vi "WPI_SerialPortWrite.vi"(8 "error in (no error)":errorcluster, 10 "Buffer":string, 11 "SerialPortRef":T1) -> (0 "error out":errorcluster, 2 "Num Bytes Written":u32, 3 "SerialPortRef":T1)   [LabVIEW 2017]
doc: "Writes data to the serial device you specify.\n\nThis software is licensed. Open the labview\\readme\\WPI Robotics Library Open Source License.txt file for more information."
uses:
  <vilib>/Rock Robotics/WPI/SerialPort/WPI_SerialPortRef.ctl
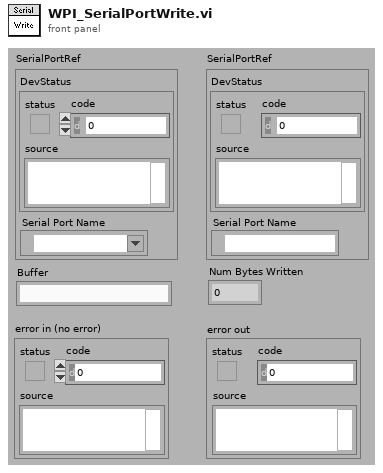
[diagram p1: front panel]
types:
  T1 = typedef "WPI_SerialPortRef.ctl" = cluster{"DevStatus":errorcluster, "Serial Port Name":refnum<visa-resource-name>}
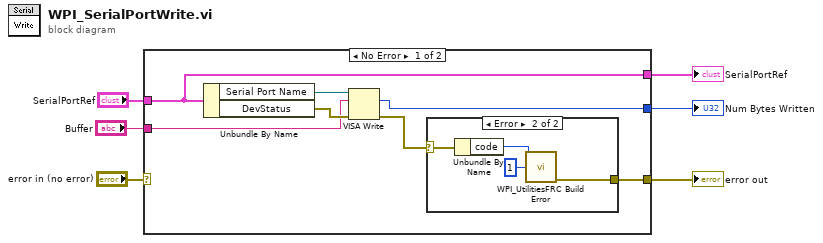
[diagram p0: block diagram]
diagram:
  n1 = case shown="No Error" "error in (no error)" {
    selector: "error in (no error)" -> [_ w20]
    tunnel: "SerialPortRef" -> [w7 w19]
    tunnel: [w7 w19] -> w5
    tunnel: [w8 w20] -> w3
    tunnel: [w11 _] -> w2
    tunnel: "Buffer" -> [w10 _]
    frame No Error {
      n2 = Unbundle By Name(w7) -> ("Serial Port Name"=w13:refnum<visa-resource-name>, "DevStatus"=w12:errorcluster)
      n3 = VISA Write(VISA resource name=w13, write buffer=w10, error in (no error)=w12) -> (return count=w11:u32, error out=w9:errorcluster)  [unwired: 1 out]
      n4 = case shown="Error" w9 {
        selector: w9 -> [w14 w16]
        tunnel: [w14 w15] -> w8
        frame No Error {
        }
        frame Error {
          n5 = Unbundle By Name(w16) -> ("code"=w18:i32)
          n6 = call <vilib>:"WPI_UtilitiesFRC Build Error.vi"("error code"=w18, "chain levels to remove (1)"=1) -> ("error out"=w15:errorcluster)  [unwired: 3 in, 10 out]
        }
      }
    }
    frame Error {
    }
  }
  "error out" <- w3
  "SerialPortRef" <- w5
  "Num Bytes Written" <- w2
